vi "ImageInitialize.vi"(8 "error in (no error)":errorcluster, 11 "Actor in":refnum<class "Actor.lvclass">) -> (0 "error out":errorcluster, 3 "Actor out":refnum<class "Actor.lvclass">)   [LabVIEW 2015, in "Actor.lvclass"]
uses:
  Actor.lvclass
  Actor.lvclass/Actor.ctl
  ImageOperaion/ImageOperation.lvclass
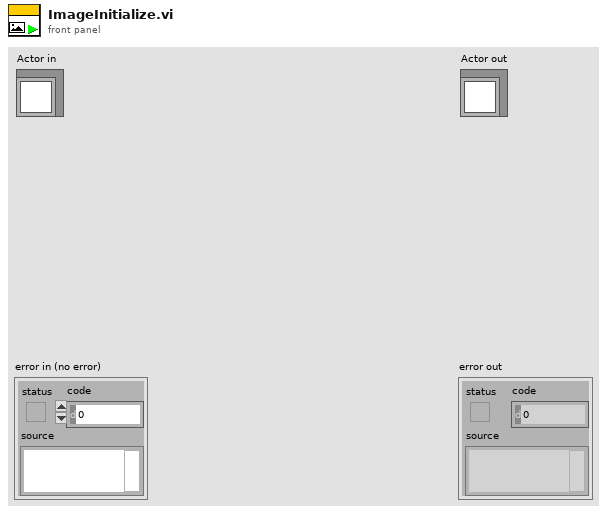
[diagram p1: front panel]
types:
  T1 = typedef "Actor.lvclass/Main Ctl and VI Refenerce.ctl" = cluster{"Size":refnum<vi>, "Save Path":refnum<vi>, "Slide":refnum<vi>, "Cut":refnum<vi>, "Previous Button":refnum<vi>, "Next Button":refnum<vi>, "This VI":refnum<vi>}
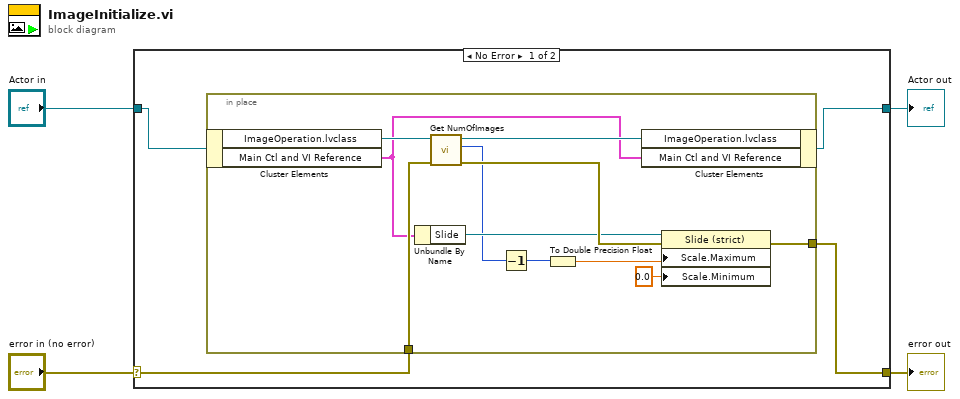
[diagram p0: block diagram]
diagram:
  n1 = case shown="No Error" "error in (no error)" {
    selector: "error in (no error)" -> [w8 w21]
    tunnel: [w7 w21] -> w3
    tunnel: [w5 w20] -> w1
    tunnel: "Actor in" -> [w6 w20]
    frame No Error {
      n2 = in-place {
        in-place-border: w8 -> [w19]
        in-place-border: [w15] -> w7
        n3 = in-place-cluster #1(w6) -> ("ImageOperation.lvclass"=w14:refnum<class "ImageOperation.lvclass">, "Main Ctl and VI Reference"=w13:T1)
        n4 = Unbundle By Name(w13) -> ("Slide"=w12:refnum<vi>)
        n5 = call "Get NumOfImages.vi"("error in (no error)"=w19, "ImageOperation in"=w14) -> ("error out"=w17:errorcluster, "NumOfImages"=w10:i32, "ImageOperation out"=w18:refnum<class "ImageOperation.lvclass">)  [unwired: 7 in]
        n6 = Decrement(x=w10) -> (x-1=w9:i32)
        n7 = To Double Precision Float(number=w9) -> (double precision float=w16:dbl)
        n8 = in-place-cluster #1("ImageOperation.lvclass"=w18, "Main Ctl and VI Reference"=w13) -> (w5:refnum<class "Actor.lvclass">)
        n9 = property class="Slide (strict)"(reference=w12, error in=w17, "Scale.Maximum"=w16, "Scale.Minimum"=0.0 ("Scale.Range:Minimum")) -> (error out=w15:errorcluster)  [unwired: 1 out]
      }
    }
    frame Error {
    }
  }
  "error out" <- w3
  "Actor out" <- w1
